vi "GetH5FileDriver.vi"(6 "error in (no error)":errorcluster, 9 "File Driver":T1) -> (0 "error out":errorcluster, 3 "HDF5 File Driver Ref out":T2)   [LabVIEW 2017]
doc: "Returns the H5 Reference for the specified file driver."
uses:
  <vilib>/UPVI/lvhdf5/library.llb/HDF5 Ref.ctl
  <vilib>/UPVI/lvhdf5/property.llb/H5FD_drivers_t.ctl
panel:
  # "LVHDF5 Toolkit\nCopyright (c) 2005-2013 by Jason D. Sommerville\nCopyright (c) 2014 by UPVI, LLC.\n\nThis use and distribution of this file is governed by the terms found in \nLICENSE.txt distributed with this toolkit and installed at\n <user.lib>\\_lvhdf5\\LICENSE.txt"
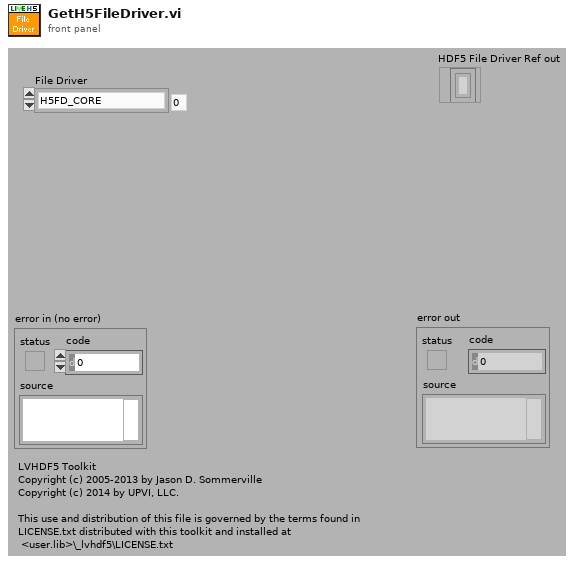
[diagram p1: front panel]
types:
  T1 = typedef "H5FD_drivers_t.ctl" = enum16{"H5FD_CORE", "H5FD_FAMILY", "H5FD_GASS", "H5FD_LOG", "H5FD_MPIO", "H5FD_MULTI", "H5FD_SEC2", "H5FD_STDIO", "H5FD_STREAM", "HF5D_DIRECT", "HF5D_WINDOWS", "H5FD_SPLIT", "H5FD_MPIPOSIX"}
  T2 = typedef "HDF5 Ref.ctl" = refnum<k1>
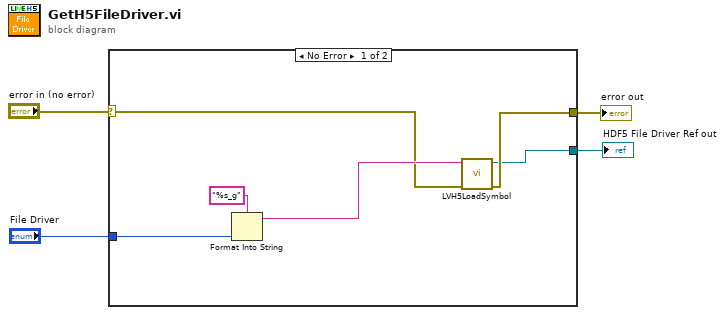
[diagram p0: block diagram]
diagram:
  n1 = case shown="No Error" "error in (no error)" {
    selector: "error in (no error)" -> [w7 w11]
    tunnel: [w6 w11] -> w3
    tunnel: "File Driver" -> [w10 _]
    tunnel: [w5 _] -> w1
    frame No Error {
      n2 = Format Into String(format string="%s_g", w10) -> (resulting string=w8:string)  [unwired: 2 in, 1 out]
      n3 = call <vilib>:"LVH5LoadSymbol.vi"("error in (no error)"=w7, "Symbol"=w8) -> ("error out"=w6:errorcluster, "Refnum out"=w5:T2)  [unwired: 8 in]
    }
    frame Error {
    }
  }
  "error out" <- w3
  "HDF5 File Driver Ref out" <- w1
